vi "set_V_one_channel.vi"() -> ()   [LabVIEW 2017]
uses:
  types/channels_enum.ctl
panel:
  in  "value_control":bool=TRUE
  out "error out":errorcluster
  out "VISA resource name 2":refnum<visa-resource-name>
  in  "voltage":dbl=0.001 min=0.0 max=120.0
  in  "channel":T1=enum."1"
  in  "error in (no error)":errorcluster
  in  "VISA resource name":refnum<visa-resource-name>
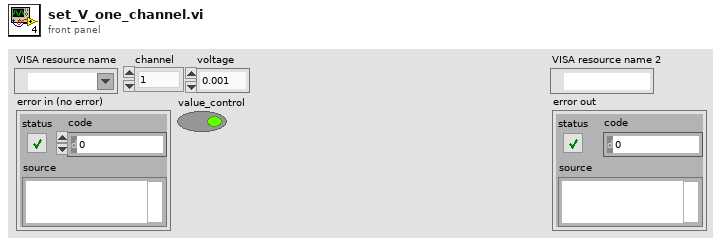
[diagram p1: front panel]
types:
  T1 = typedef "channels_enum.ctl" = enum16{"0", "1", "2"}
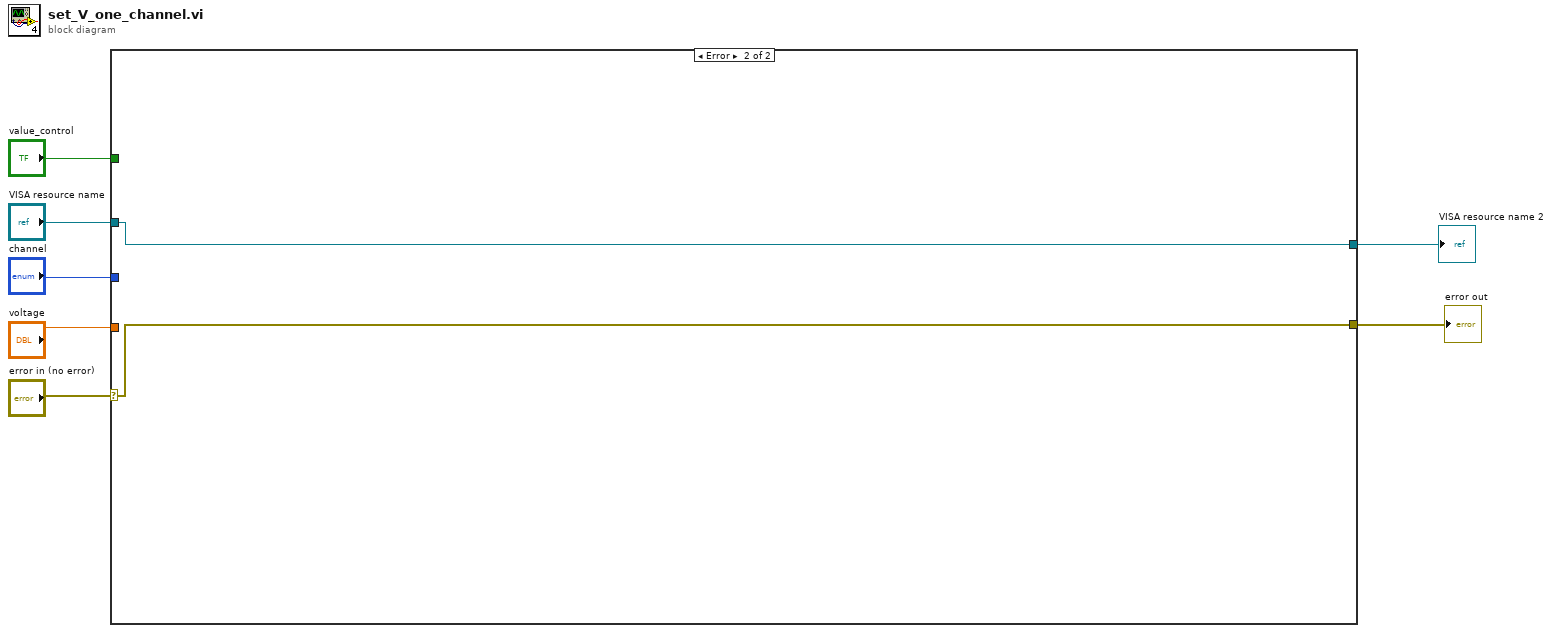
[diagram p0: block diagram]
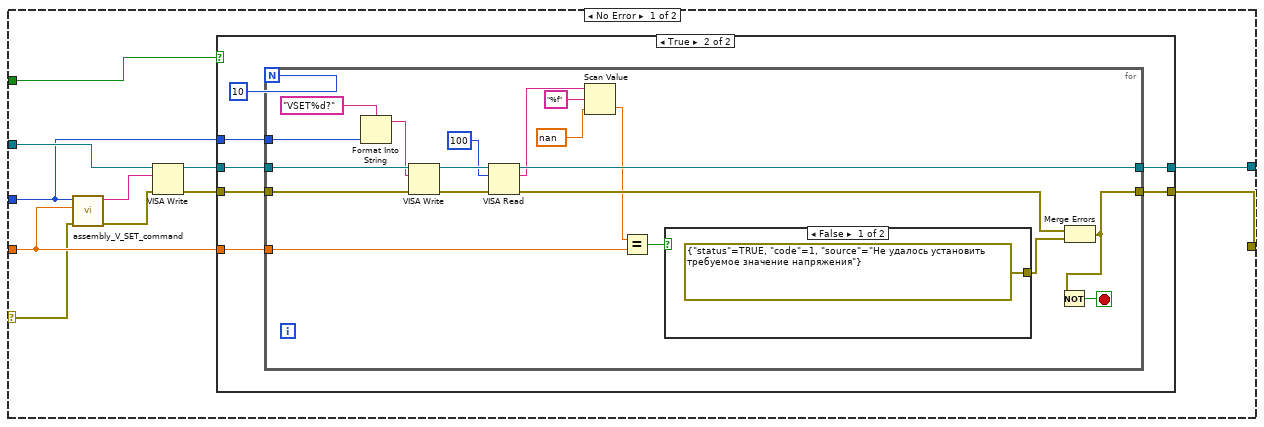
[diagram p2: hidden frame]
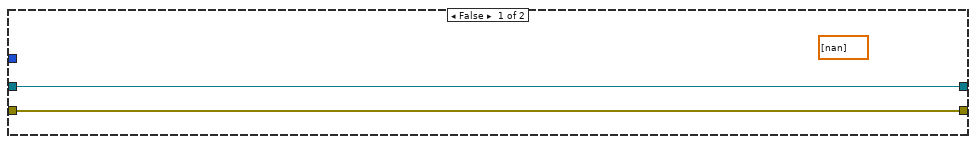
[diagram p3: hidden frame]
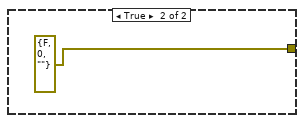
[diagram p4: hidden frame]
diagram:
  n1 = case shown="Error" "error in (no error)" {
    selector: "error in (no error)" -> [w8 w50]
    tunnel: "VISA resource name" -> [w18 w49]
    tunnel: [w15 w49] -> w6
    tunnel: [w14 w50] -> w5
    tunnel: "value_control" -> [w13 _]
    tunnel: "channel" -> [w11 _]
    tunnel: "voltage" -> [w10 _]
    frame No Error {
      n2 = call "assembly_V_SET_command.vi"("error_in"=w8, "voltage"=w10, "channel"=w11) -> ("error_out"=w9:errorcluster, "command"=w12:string)  [unwired: 7 in]
      n3 = VISA Write(VISA resource name=w18, write buffer=w12, error in (no error)=w9) -> (VISA resource name out=w17:refnum<visa-resource-name>, error out=w16:errorcluster)  [unwired: 1 out]
      n4 = case shown="True" w13 {
        tunnel: w17 -> [w20 w27]
        tunnel: w16 -> [w19 w26]
        tunnel: [w20 w24] -> w15
        tunnel: [w19 w23] -> w14
        tunnel: w10 -> [_ w22]
        tunnel: w11 -> [_ w21]
        frame False {
          (unwired) dbl[] [nan]
        }
        frame True {
          n5 = for {
            N: 10 -> [_]
            tunnel: w27 -> [w46]
            tunnel: w26 -> [w45]
            tunnel: [w41] -> w24
            tunnel: [w33] -> w23
            tunnel: w22 -> [w37]
            tunnel: w21 -> [w30]
            stop <- w34 stop-if-true
            n6 = Format Into String(format string="VSET%d?" ("write buffer"), w30) -> (resulting string=w28:string)  [unwired: 2 in, 1 out]
            n7 = VISA Write(VISA resource name=w46, write buffer=w28, error in (no error)=w45) -> (VISA resource name out=w44:refnum<visa-resource-name>, error out=w43:errorcluster)  [unwired: 1 out]
            n8 = VISA Read(VISA resource name=w44, byte count=u32 100, error in (no error)=w43) -> (VISA resource name out=w41:refnum<visa-resource-name>, read buffer=w39:string, error out=w35:errorcluster)  [unwired: 1 out]
            n9 = Scan Value(string=w39, format string="%f", default (0 dbl)=nan) -> (value=w31:dbl)  [unwired: 1 out]
            n10 = Equal?(x=w31, y=w37) -> (x = y?=w38:bool)
            n11 = case shown="False" w38 {
              tunnel: [errorcluster {"status"=TRUE, "code"=1, "source"="Не удалось установить требуемое значение напряжения"} ("error constant") errorcluster {"status"=FALSE, "code"=0, "source"=""} ("error constant")] -> w36
              frame False {
              }
              frame True {
              }
            }
            n12 = Merge Errors(w35, w36) -> (w33:errorcluster)
            n13 = Not(x=w33) -> (.not. x?=w34:bool)
          }
        }
      }
    }
    frame Error {
    }
  }
  "VISA resource name 2" <- w6
  "error out" <- w5
